vi "GetUserInformation.vi"(8 "error in (no error)":errorcluster, 10 "UserInfo":string, 11 "UserManagement in":refnum<class "UserManagement.lvclass">) -> (0 "error out":errorcluster, 3 "UserManagement out":refnum<class "UserManagement.lvclass">)   [LabVIEW 2019, in "UserManagement.lvlib" / "UserManagement.lvclass"]
uses:
  UserManagement.lvclass
  User.ctl
  Permission.ctl
  UserManagement.lvclass/UserManagement.ctl
  <vilib>/Utility/config.llb/Read Key (String).vi
  <vilib>/Utility/config.llb/NI_LVConfig.lvlib
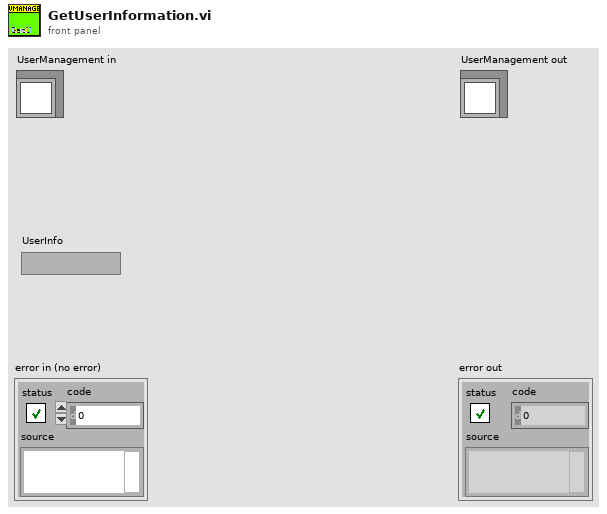
[diagram p1: front panel]
types:
  T1 = typedef "UserManagement.lvlib/UserManagement.lvclass/User.ctl" = cluster{"Permission":T2, "UserName":string, "PassWord":string}
  T2 = typedef "UserManagement.lvlib/UserManagement.lvclass/Permission.ctl" = enum16{"Engineer", "Technical", "Operator"}
  T3 = cluster{"Enginner":T1[], "Technical":T1[], "Operator":T1[]}
  T4 = typedef "NI_LVConfig.lvlib/Config Data RefNum.ctl" = refnum<k1>
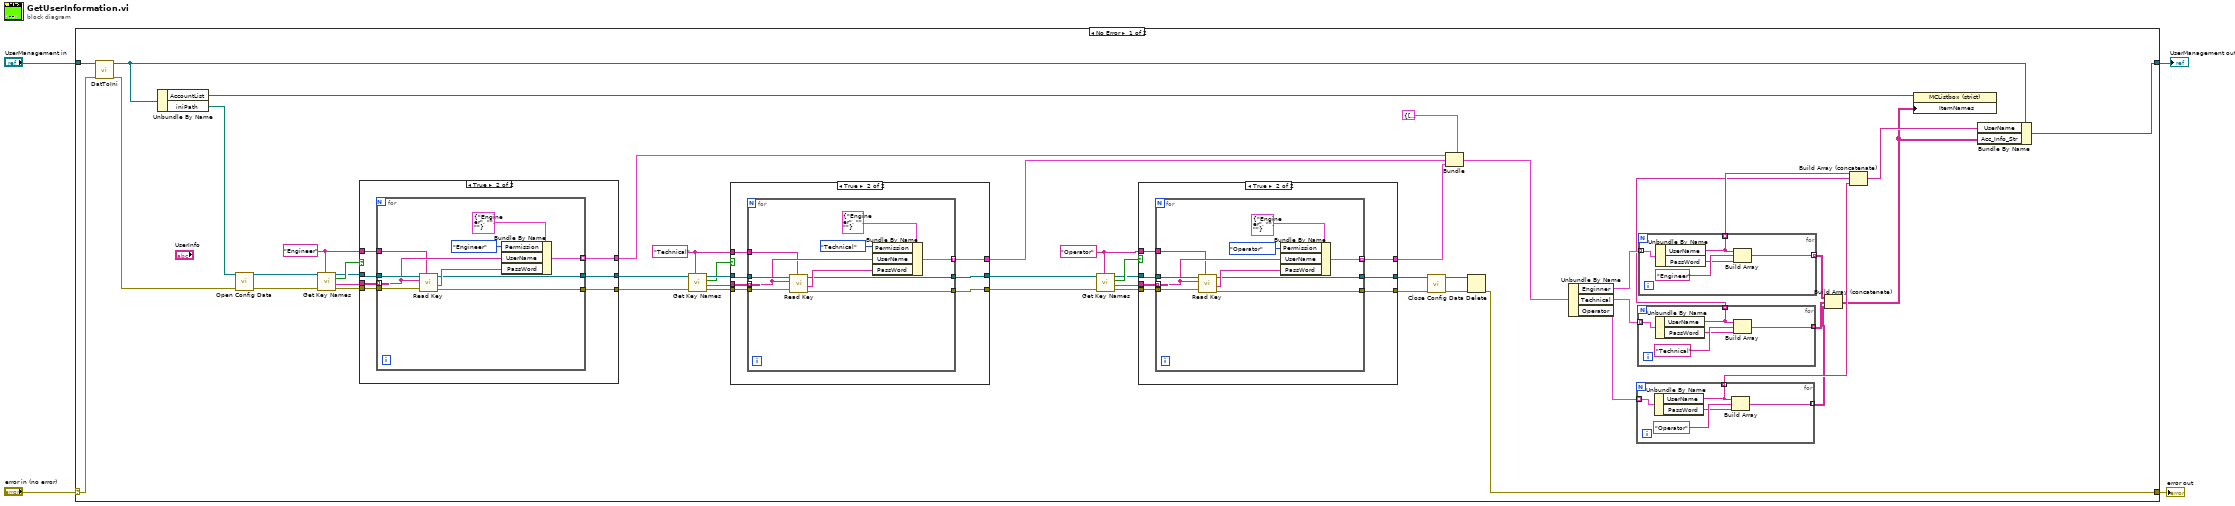
[diagram p0: block diagram]
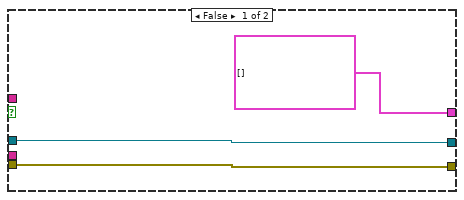
[diagram p2: hidden frame]
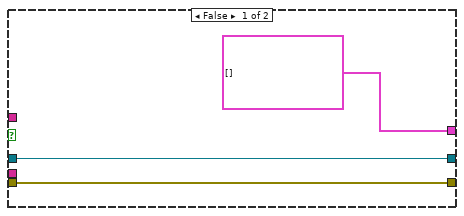
[diagram p3: hidden frame]
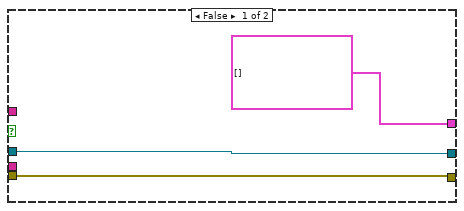
[diagram p4: hidden frame]
diagram:
  n1 = case shown="No Error" "error in (no error)" {
    selector: "error in (no error)" -> [w6 w130]
    tunnel: [w24 w130] -> w3
    tunnel: [w12 w129] -> w1
    tunnel: "UserManagement in" -> [w8 w129]
    frame No Error {
      w28 = "Operator" ("section")
      w29 = "Technical" ("section")
      w30 = "Engineer" ("section")
      n2 = call-dynamic "DatToIni.vi"("error in (no error)"=w6, "UserManagement in"=w8) -> ("error out"=w5:errorcluster, "UserManagement out"=w7:refnum<class "UserManagement.lvclass">)  [unwired: 8 in]
      n3 = Unbundle By Name(w7) -> ("AccountList"=w10:refnum<vi>, "iniPath"=w27:path)
      n4 = call <vilib>:"Open Config Data.vi"("error in (no error)"=w5, "configuration file path"=w27) -> ("error out"=w52:errorcluster, "refnum"=w53:T4)  [unwired: 7 in, 1 out]
      n5 = call <vilib>:"Get Key Names.vi"("section"=w30, "error in (no error)"=w52, "refnum"=w53) -> ("error out"=w51:errorcluster, "key names"=w48:string[], "section exists?"=w50:bool, "refnum out"=w49:T4)  [unwired: 5 in]
      n6 = case shown="True" w50 {
        tunnel: w51 -> [w110 w117]
        tunnel: w49 -> [w109 w116]
        tunnel: w48 -> [_ w118]
        tunnel: [T1[] [] w115] -> w35
        tunnel: [w110 w114] -> w42
        tunnel: [w109 w113] -> w43
        tunnel: w30 -> [_ w112]
        frame False {
        }
        frame True {
          n7 = for {
            tunnel: w118 -> [w126] mode=indexing
            tunnel: w117 -> [w127]
            tunnel: w116 -> [w128]
            tunnel: [w124] -> w115 mode=indexing
            tunnel: [w123] -> w114
            tunnel: [w122] -> w113
            tunnel: w112 -> [w121]
            n8 = call-poly <vilib>:"Read Key.vi"("section"=w121, "error in (no error)"=w127, "key"=w126, "refnum"=w128) -> ("error out"=w123:errorcluster, "value"=w125:string, "refnum out"=w122:T4)  [unwired: 4 in, 1 out]
            n9 = Bundle By Name(cluster=T1 {"Permission"=enum."Engineer", "UserName"="", "PassWord"=""} ("User"), "Permission"=Permission."Engineer", "UserName"=w126, "PassWord"=w125) -> (w124:T1)
          }
        }
      }
      n10 = call <vilib>:"Get Key Names.vi"("section"=w29, "error in (no error)"=w42, "refnum"=w43) -> ("error out"=w44:errorcluster, "key names"=w47:string[], "section exists?"=w45:bool, "refnum out"=w46:T4)  [unwired: 5 in]
      n11 = case shown="True" w45 {
        tunnel: w44 -> [w91 w97]
        tunnel: w46 -> [w90 w96]
        tunnel: w47 -> [_ w98]
        tunnel: [T1[] [] w95] -> w34
        tunnel: [w91 w94] -> w36
        tunnel: [w90 w93] -> w37
        tunnel: w29 -> [_ w92]
        frame False {
        }
        frame True {
          n12 = for {
            tunnel: w98 -> [w106] mode=indexing
            tunnel: w97 -> [w107]
            tunnel: w96 -> [w108]
            tunnel: [w104] -> w95 mode=indexing
            tunnel: [w103] -> w94
            tunnel: [w102] -> w93
            tunnel: w92 -> [w101]
            n13 = call-poly <vilib>:"Read Key.vi"("section"=w101, "error in (no error)"=w107, "key"=w106, "refnum"=w108) -> ("error out"=w103:errorcluster, "value"=w105:string, "refnum out"=w102:T4)  [unwired: 4 in, 1 out]
            n14 = Bundle By Name(cluster=T1 {"Permission"=enum."Engineer", "UserName"="", "PassWord"=""} ("User"), "Permission"=Permission."Technical", "UserName"=w106, "PassWord"=w105) -> (w104:T1)
          }
        }
      }
      n15 = call <vilib>:"Get Key Names.vi"("section"=w28, "error in (no error)"=w36, "refnum"=w37) -> ("error out"=w41:errorcluster, "key names"=w38:string[], "section exists?"=w40:bool, "refnum out"=w39:T4)  [unwired: 5 in]
      n16 = case shown="True" w40 {
        tunnel: w41 -> [w71 w77]
        tunnel: w39 -> [w70 w76]
        tunnel: w38 -> [_ w78]
        tunnel: [T1[] [] w75] -> w33
        tunnel: [w71 w74] -> w31
        tunnel: [w70 w73] -> w32
        tunnel: w28 -> [_ w72]
        frame False {
        }
        frame True {
          n17 = for {
            tunnel: w78 -> [w86] mode=indexing
            tunnel: w77 -> [w87]
            tunnel: w76 -> [w88]
            tunnel: [w84] -> w75 mode=indexing
            tunnel: [w83] -> w74
            tunnel: [w82] -> w73
            tunnel: w72 -> [w81]
            n18 = call-poly <vilib>:"Read Key.vi"("section"=w81, "error in (no error)"=w87, "key"=w86, "refnum"=w88) -> ("error out"=w83:errorcluster, "value"=w85:string, "refnum out"=w82:T4)  [unwired: 4 in, 1 out]
            n19 = Bundle By Name(cluster=T1 {"Permission"=enum."Engineer", "UserName"="", "PassWord"=""} ("User"), "Permission"=Permission."Operator", "UserName"=w86, "PassWord"=w85) -> (w84:T1)
          }
        }
      }
      n20 = call <vilib>:"Close Config Data.vi"("error in (no error)"=w31, "refnum"=w32) -> ("error out"=w25:errorcluster, "file path"=w26:path)  [unwired: 8 in]
      n21 = Bundle(cluster=T3 {"Enginner"=[], "Technical"=[], "Operator"=[]} ("Cluster 2"), "Enginner"=w35, "Technical"=w34, "Operator"=w33) -> (w13:T3)
      n22 = Delete(path (use dialog)=w26, error in=w25) -> (error out=w24:errorcluster)  [unwired: 3 in, 2 out]
      n23 = Unbundle By Name(w13) -> ("Enginner"=w23:T1[], "Technical"=w22:T1[], "Operator"=w17:T1[])
      n24 = for {
        tunnel: w17 -> [w58] mode=indexing
        tunnel: [w56] -> w15 mode=indexing
        tunnel: [w54] -> w16 mode=indexing
        n25 = Unbundle By Name(w58) -> ("UserName"=w54:string, "PassWord"=w55:string)
        n26 = Build Array(w54, "Operator", w55) -> (w56:string[])
      }
      n27 = for {
        tunnel: w22 -> [w63] mode=indexing
        tunnel: [w61] -> w20 mode=indexing
        tunnel: [w59] -> w18 mode=indexing
        n28 = Unbundle By Name(w63) -> ("UserName"=w59:string, "PassWord"=w60:string)
        n29 = Build Array(w59, "Technical", w60) -> (w61:string[])
      }
      n30 = for {
        tunnel: w23 -> [w68] mode=indexing
        tunnel: [w66] -> w21 mode=indexing
        tunnel: [w64] -> w19 mode=indexing
        n31 = Unbundle By Name(w68) -> ("UserName"=w64:string, "PassWord"=w65:string)
        n32 = Build Array(w64, "Engineer", w65) -> (w66:string[])
      }
      n33 = Build Array (concatenate)(w21, w20, w15) -> (w9:string[][])
      n34 = Build Array (concatenate)(w19, w18, w16) -> (w11:string[])
      n35 = property class="MCListbox (strict)"(reference=w10, "ItemNames"=w9) -> ()  [unwired: 1 in, 2 out]
      n36 = Bundle By Name(cluster=w7, "UserName"=w11, "Acc_Info_Str"=w9) -> (w12:refnum<class "UserManagement.lvclass">)
    }
    frame Error {
    }
  }
  "error out" <- w3
  "UserManagement out" <- w1
